vi "global-GEvnt Filter Change Flag.vi"() -> ()   [LabVIEW 2017, in "Communicable State Machine.lvlib"]
doc: "### global-GEvnt Filter Change Flag.vi\n\nGlobal variable used to indicate whether the Global Event filter conditions have changed"
uses:
  Communicable State Machine.lvlib
panel:
  in  "global-GEvnt Filter Change Flag":u64=4603270806574966694 format="%08x"
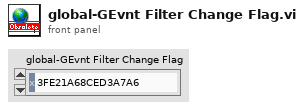
[diagram p1: front panel]
diagram:
